vi "is_not_missclick.vi"(11 "input":cluster{i32, i32, i32, i32}) -> (3 "notMissclick":bool)   [LabVIEW 2021]
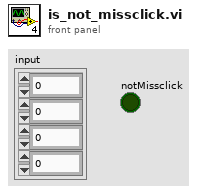
[diagram p1: front panel]
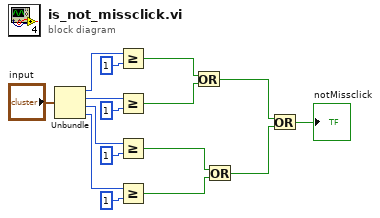
[diagram p0: block diagram]
diagram:
  n1 = Unbundle("input") -> (w16:i32, w13:i32, w11:i32, w9:i32)
  n2 = Greater Or Equal?(x=w16, y=1) -> (x >= y?=w8:bool)
  n3 = Greater Or Equal?(x=w13, y=1) -> (x >= y?=w7:bool)
  n4 = Greater Or Equal?(x=w11, y=1) -> (x >= y?=w6:bool)
  n5 = Greater Or Equal?(x=w9, y=1) -> (x >= y?=w5:bool)
  n6 = Or(x=w8, y=w7) -> (x .or. y?=w4:bool)
  n7 = Or(x=w6, y=w5) -> (x .or. y?=w3:bool)
  n8 = Or(x=w4, y=w3) -> (x .or. y?=→"notMissclick":bool)
